vi "Main Loop.vi"(8 "error in (no error)":errorcluster, 10 "Chart Notifier":refnum<notifier>, 11 "Message Queues":T1) -> (0 "error out":errorcluster)   [LabVIEW 2018, in "Pump Module.lvlib" / "Pump Module Engine.lvlib"]
uses:
  Pump Module Engine.lvlib
  All Message Queues.ctl
  support/Message Queue/Message Cluster.ctl
  State Cluster.ctl
  State Enum.ctl
  Pump Module Settings Cluster.ctl
  Measure Instrument/PID 2 Output Enum.ctl
  Ismatec ISM 831C/Controls/Ismatech ISM831C Settings Cluster.ctl
  Ismatec 78001/Ismatec 4083.ctl
  Masterflex 7550-30/Controls/Settings Cluster.ctl
  VICI M50 Party Mode/Settings Cluster.ctl
  Tacmina QI/Tacmina QI DAQ Setting.ctl
  KNF Pump/Settings Cluster plus SIMDOS.ctl
  ASIA Pump/Pump Settings.ctl
  FLOM Pump/Settings Cluster.ctl
  SSI PR Class/SSI PR or LD Settings Cluster.ctl
  Masterflex 75211/Masterflex 75211 DAQ Setting.ctl
  Pump Module Display.ctl
  <vilib>/Platform/TimedLoop/XDataNode/timing_clust.ctl
  <vilib>/Platform/TimedLoop/XDataNode/nitl_modes.ctl
  <vilib>/Platform/TimedLoop/XDataNode/wakeup.ctl
  Tag VIs/Tag FGV Operation Enum.ctl
  support/Message Queue/Enqueue Message (Single).vi
  <vilib>/Platform/TimedLoop/XDataNode/XDataNode.xnode
  support/Message Queue/Message Queue.lvlib
  <vilib>/Platform/TimedLoop/XDataNode/XDNodeRunTimeDep.lvlib
  Pump Module.lvlib
  Ismatec ISM 831C/Ismatec ISM 831C.lvlib
  Masterflex 7550-30/Masterflex 7550-30.lvlib
  Shared Variables/Dynamic Shared Variables.lvlib
  Tacmina QI/Tacmina QI.lvlib
  KNF Pump/KNF SIMDOS.lvlib
  ASIA Pump.lvlib
  VICI M50 Party Mode/VICI M6 M50 Party Mode.lvlib
  FLOM Pump/FLOM Pump.lvlib
  SSI PR Class/SSI PR or LD Pump.lvlib
  support/Support Library.lvlib
  Masterflex 75211/Masterflex 75211.lvlib
  Ismatec 78001/Ismatec 4308.lvlib
  Program Files (x86)/Pfizer/FAST/data/AsiaPumpInterface.dll
panel:
  out "error out 2":errorcluster
  out "Period (s)":dbl format="%_4g"
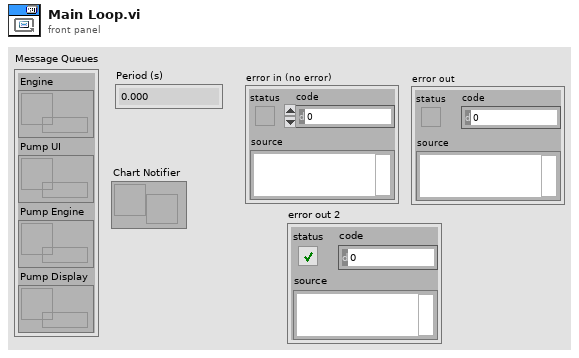
[diagram p1: front panel]
types:
  T1 = typedef "Pump Module.lvlib/All Message Queues.ctl" = cluster{"Engine":refnum<queue>, "Pump UI":refnum<queue>, "Pump Engine":refnum<queue>, "Pump Display":refnum<queue>}
  T2 = typedef "Pump Module.lvlib/Pump Module Display.ctl" = cluster{"Pump On?":enum16{"Off", "On", "Not Initialized"}, "Cycle Period":dbl, "Current Pump Speed":dbl, "Current Pump Pressure":dbl, "Current Pump Flow":dbl, "Totalized":dbl, "Output":T3}
  T3 = typedef "PID 2 Output Enum.ctl" = enum16{"Default", "Ismatec ISM 4308", "Ismatec ISM 831C", "Masterflex 7550-30", "VICI M6", "VICI M50", "Tacmina QI", "KNF SIMDOS", "ASIA Type C", "FLOM UI-22-11", "SSI PR/LD", "SSI P40", "Masterflex 75211-70"}
  T4 = typedef "XDNodeRunTimeDep.lvlib/timing_clust.ctl" = cluster{"Expected End [f-1]":u64, "Actual End [f-1]":u64, "Finished Late? [f-1]":bool, "Expected End [i-1]":u64, "Actual End [i-1]":u64, "Finished Late? [i-1]":bool, "Expected Start [i]":u64, "Actual Start [i]":u64, "Expected Start [f]":u64, "Actual Start [f]":u64, "Source Name":string, "Structure Name":string, "Period":i64, "Deadline":i64, "Offset":i64, "Start":i64, "Priority":i32, "Timeout":i32, "Mode":T5, "Wakeup Reason":T6, "Error":errorcluster, "Source Type":string, "Secondary Source Type":string, "Global End Time":u64, "Global Start Time":u64, "Frame Duration":u64, "Iteration Duration":u64, "Assigned CPU":i32, "I/O Scan Engine Mode":u32}
  T5 = typedef "XDNodeRunTimeDep.lvlib/nitl_modes.ctl" = enum32{"No Change", "Process missed periods, maintain original phase", "Discard missed periods, maintain original phase", "Process missed periods, ignore original phase", "Discard missed periods, ignore original phase"}
  T6 = typedef "XDNodeRunTimeDep.lvlib/wakeup.ctl" = enum32{"Normal", "Aborted", "Asynchronous wakeup", "Timing source error", "Timed loop error", "Timeout"}
  T7 = cluster{"enable? (F)":bool, "name":string, "alarm on":bool, "priority":u32, "ack type":enum16{"Auto", "User", "None", "Each Occurrence"}, "area":string, "description":string, "log? (T)":bool}
  T8 = typedef "Tag FGV Operation Enum.ctl" = enum16{"Init", "Set Notification Queue", "Create Tag", "Commit", "Write Tag (Numeric)", "Write Tag (Boolean)", "Read All Tags", "Read One Tag", "Delete Tag Category", "Set Alarm Parameters (Numeric)", "Set Alarm Parameters (Boolean)", "Enable All Alarms", "Disable All Alarms", "Delete All Tags", "Read Alarms", "Ack Alarm", "Read Alarm Parameters (Numeric)", "Read Alarm Parameters (Boolean)"}
  T9 = enum32{"u32BitField", "bool", "double", "string", "int8", "uint8", "int16", "uint16", "int32", "uint32", "int64", "uint64", "single", "double waveform", "int16 waveform", "array of boolean", "array of int8", "array of uint8", "array of int16", "array of uint16", "array of int32", "array of uint32", "array of int64", "array of uint64", "array of single", "array of double", "array of double waveform", "array of int16 waveform", "array of string", "variant", "timestamp", "fixed point", "custom"}
  T10 = typedef "Pump Module.lvlib/Pump Module Engine.lvlib/State Enum.ctl" = enum16{"Measuring", "Idle", "Paused"}
  T11 = typedef "Pump Module.lvlib/Pump Module Engine.lvlib/State Cluster.ctl" = cluster{"State":T10, "Start Time":timestamp, "Configuration":T12, "Current Time":timestamp, "First Iteration":bool, "Data":cluster{"Pump Speed":dbl, "Pump Pressure":dbl, "Pump Flow":dbl, "Totalized":dbl}, "Process Name":string, "Pump On?":enum16{"Off", "On", "Not Initialized"}, "Output Error":bool, "Log Started":bool, "Overpressure Alarming":bool}
  T12 = typedef "Pump Module.lvlib/Pump Module Settings Cluster.ctl" = cluster{"Cycle Period":dbl, "Manual Entry":dbl, "Output Device":T3, "Ismatech":T13, "Ismatech 3 Channel Settings":T14, "Masterflex":T15, "VICI Settings":T16, "Tacmina Settings":T17, "KNF SIMDOS Settings":T18, "ASIA Pump C":T19, "FLOM Settings":T20, "SSI PR/LD Settings":T21, "SSI P40 Settings":T21, "Masterflex 75211 Settings":T22, "Pump Calibration File":path, "Calibration Slope":dbl, "Calibration Y Intercept":dbl, "Pump Cal Enum":u16, "Reset Totalizer":bool}
  T13 = typedef "Ismatec ISM 831C.lvlib/Ismatech ISM831C Settings Cluster.ctl" = cluster{"VISA resource name":refnum<visa-resource-name>, "Simulated?":bool, "Pump Number":dbl, "Reverse?":bool}
  T14 = typedef "Ismatec 4308.lvlib/Ismatec 4083.ctl" = cluster{"VISA resource name":refnum<visa-resource-name>, "Pump Number":i16, "Channel Number":i16, "Simulated?":bool, "Reverse?":bool}
  T15 = typedef "Masterflex 7550-30.lvlib/Settings Cluster.ctl" = cluster{"VISA resource name":refnum<visa-resource-name>, "Simulated?":bool, "Pump Number":dbl, "Reverse?":bool}
  T16 = typedef "VICI M6 M50 Party Mode.lvlib/Settings Cluster.ctl" = cluster{"VISA resource name":refnum<visa-resource-name>, "Pump ID":string, "Pump Head Vol":dbl, "Reverse?":bool, "Simulated?":bool}
  T17 = typedef "Tacmina QI.lvlib/Tacmina QI DAQ Setting.ctl" = cluster{"Analog DAQ Task":refnum<k21>, "Digital DAQ Task":refnum<k21>}
  T18 = typedef "KNF SIMDOS.lvlib/Settings Cluster plus SIMDOS.ctl" = cluster{"VISA resource name":refnum<visa-resource-name>, "Simulated?":bool}
  T19 = typedef "ASIA Pump.lvlib/Pump Settings.ctl" = cluster{"ASIA Pump #":i32, "channel":i32, "Simulated":bool}
  T20 = typedef "FLOM Pump.lvlib/Settings Cluster.ctl" = cluster{"VISA resource name":refnum<visa-resource-name>, "Simulated?":bool, "Pump Number":dbl}
  T21 = typedef "SSI PR or LD Pump.lvlib/SSI PR or LD Settings Cluster.ctl" = cluster{"VISA resource name":refnum<visa-resource-name>, "Simulated?":bool}
  T22 = typedef "Masterflex 75211.lvlib/Masterflex 75211 DAQ Setting.ctl" = cluster{"Analog DAQ Task":refnum<k21>, "Digital DAQ Task":refnum<k21>}
  T23 = enum16{"Error", "Uninitialised", "Initialising", "Idle", "Filling", "Full", "Emptying", "Empty", "Pumping", "Default"}
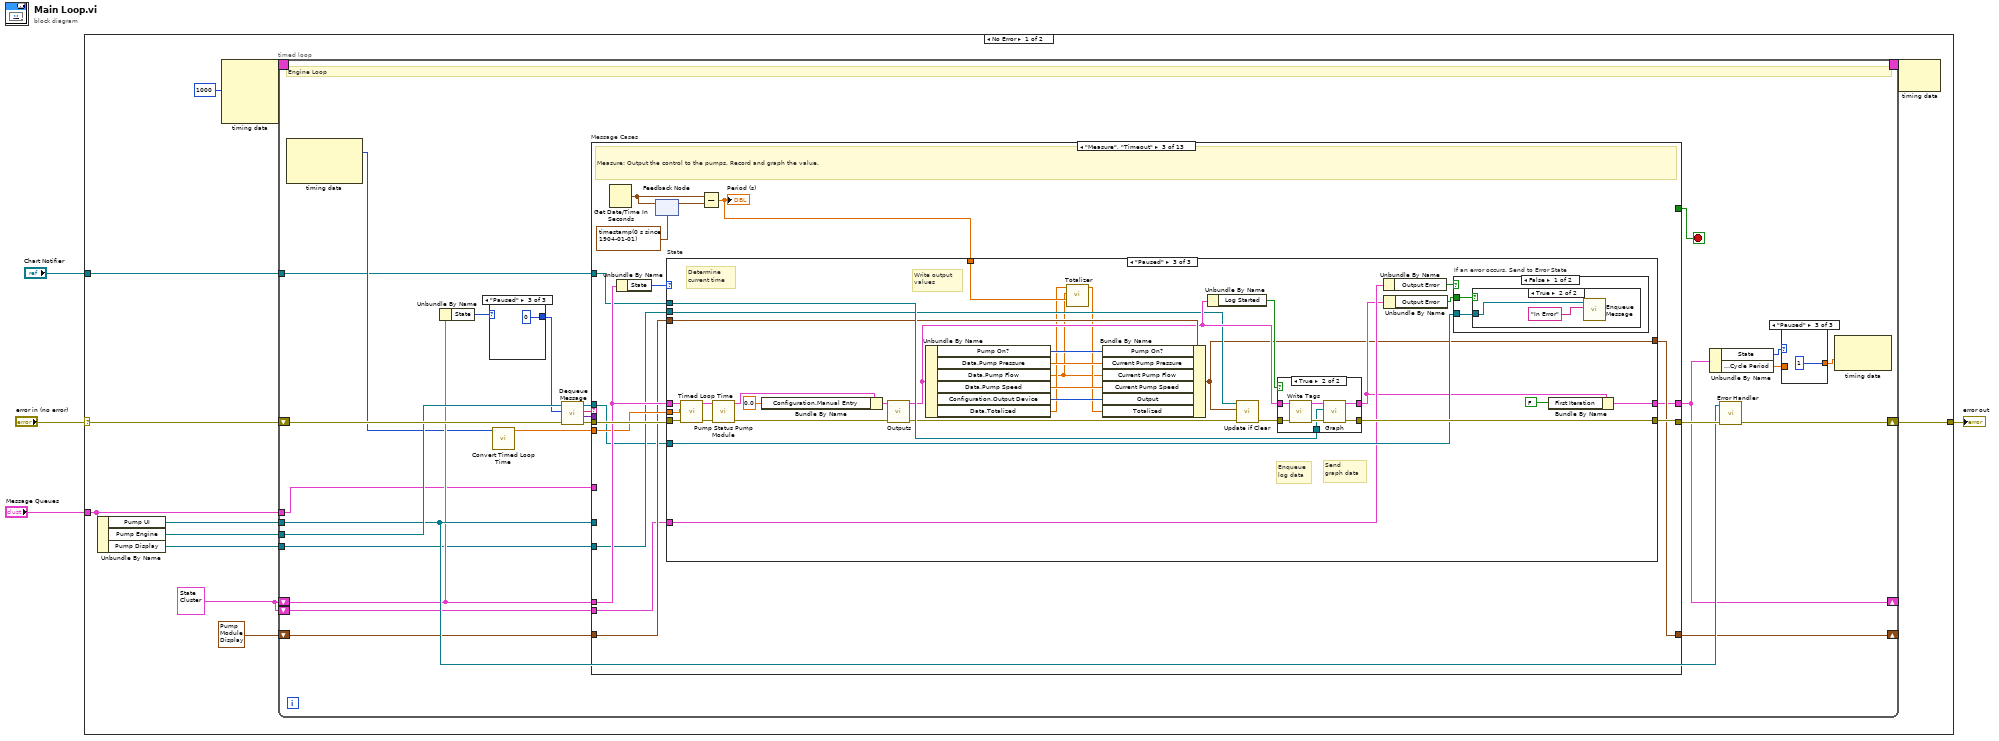
[diagram p0: block diagram]
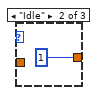
[diagram p3: hidden frame]
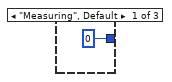
[diagram p4: hidden frame]
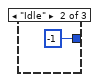
[diagram p5: hidden frame]
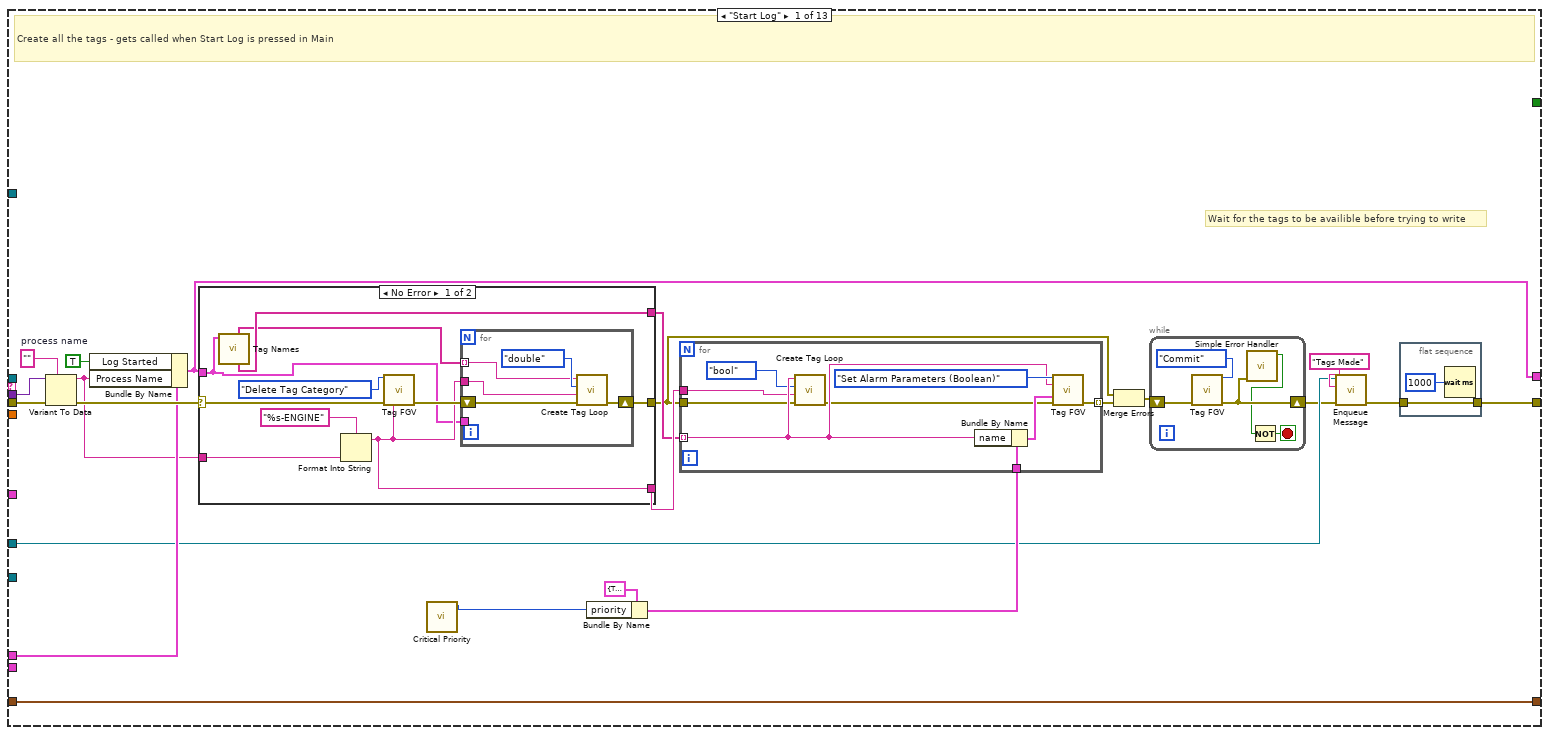
[diagram p6: hidden frame]
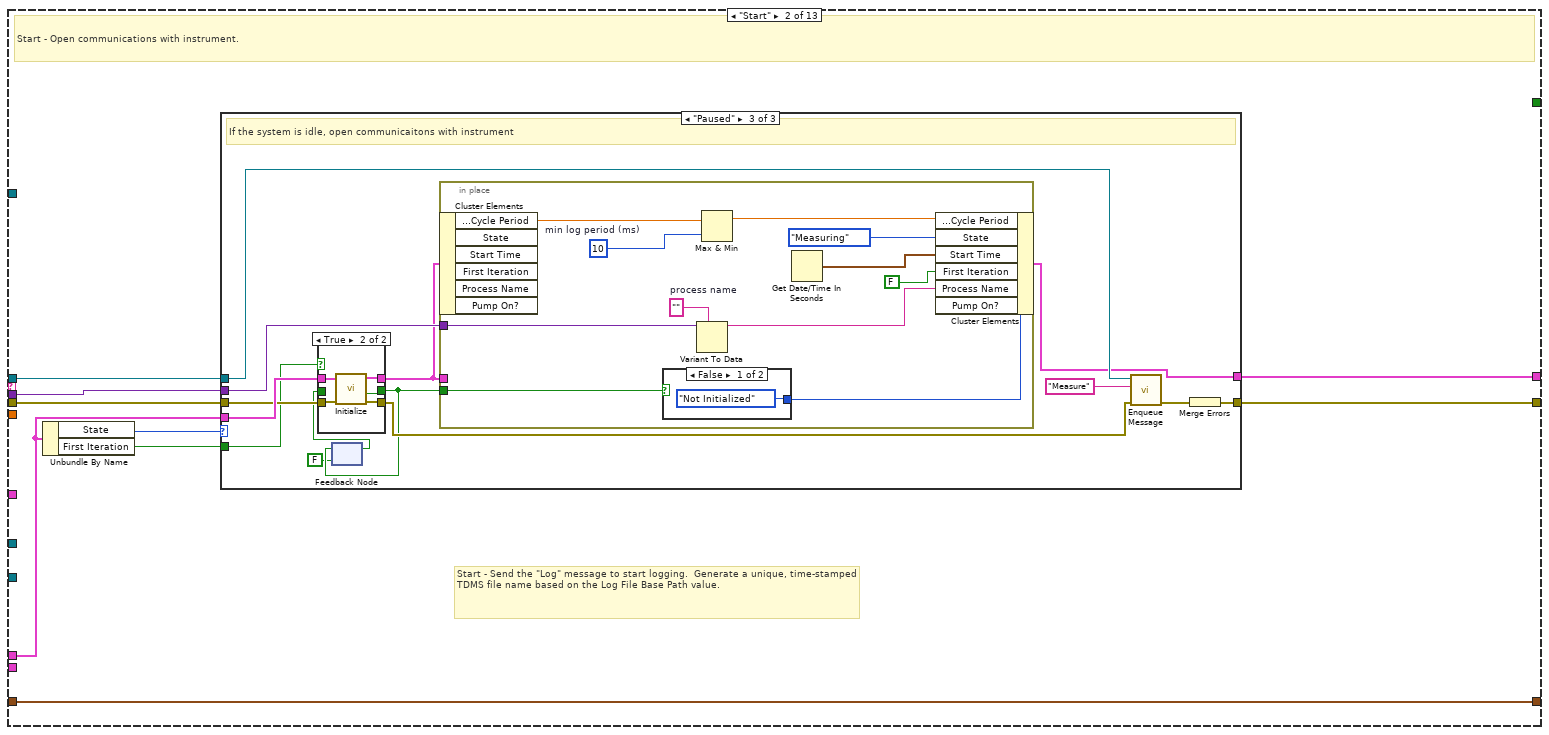
[diagram p8: hidden frame]
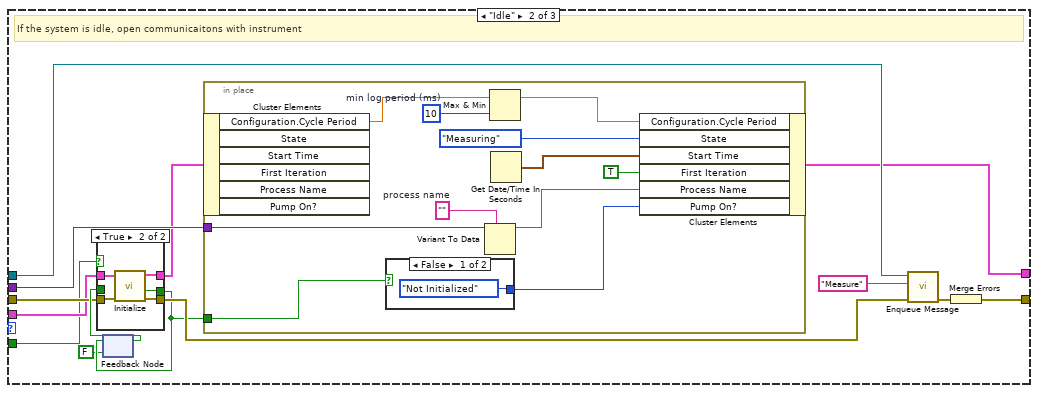
[diagram p10: hidden frame]
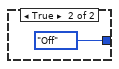
[diagram p11: hidden frame]
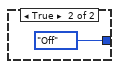
[diagram p13: hidden frame]
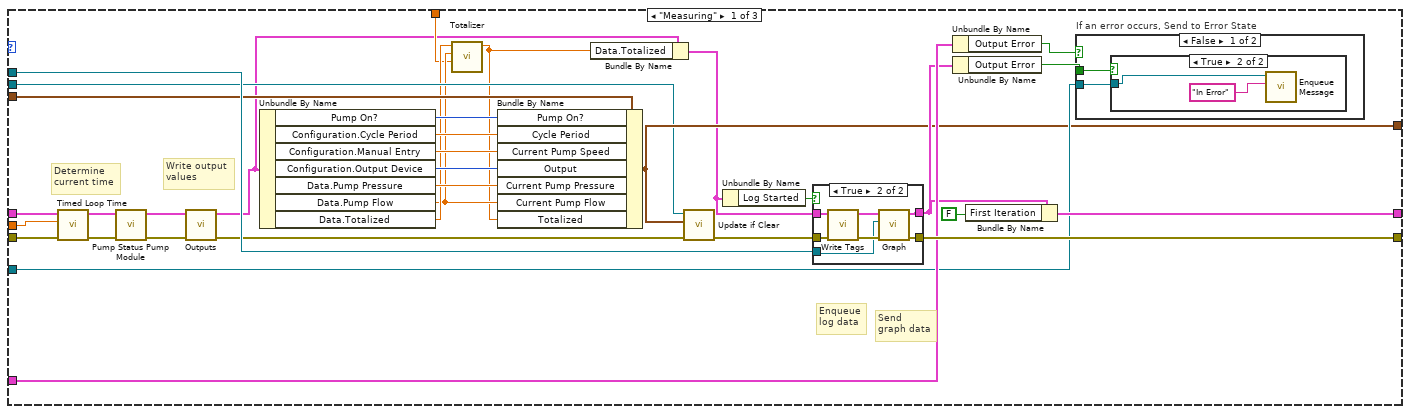
[diagram p15: hidden frame]
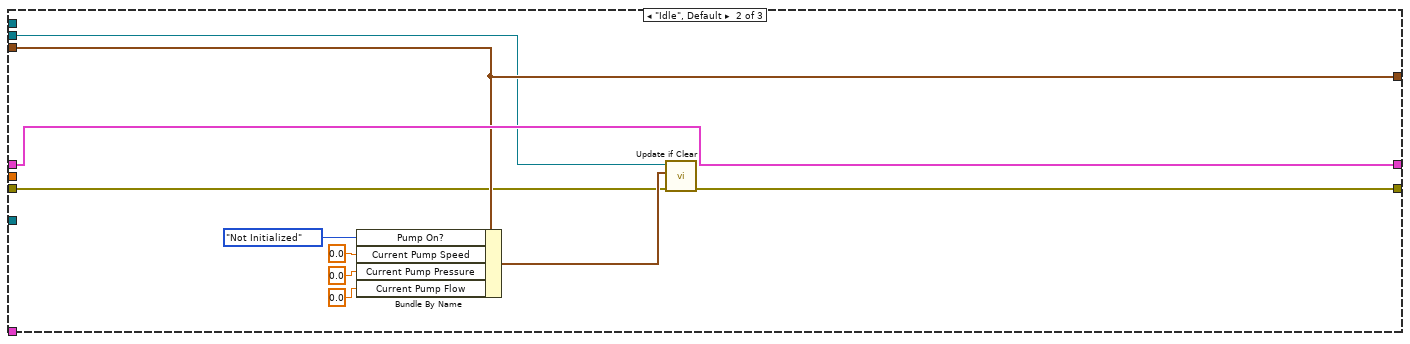
[diagram p19: hidden frame]
diagram:
  n1 = case shown="No Error" "error in (no error)" {
    selector: "error in (no error)" -> [w15 w512]
    tunnel: "Message Queues" -> [w11 _]
    tunnel: [w16 w512] -> w3
    tunnel: "Chart Notifier" -> [w9 _]
    frame No Error {
      w6 = T11 {"State"=enum."Idle", "Start Time"=timestamp(0 s since 1904-01-01), "Configuration"={"Cycle Period"=0.0, "Manual Entry"=0.0, "Output Device"=enum."VICI M6", "Ismatech"={"VISA resource name"="", "Simulated?"=FALSE, "Pump Number"=1.0, "Reverse?"=FALSE}, "Ismatech 3 Channel Settings"={"VISA resource name"="", "Pump Number"=1, "Channel Number"=0, "Simulated?"=TRUE, "Reverse?"=FALSE}, "Masterflex"={"VISA resource name"="", "Simulated?"=FALSE, "Pump Number"=1.0, "Reverse?"=FALSE}, "VICI Settings"={"VISA resource name"="", "Pump ID"="", "Pump Head Vol"=0.0, "Reverse?"=FALSE, "Simulated?"=FALSE}, "Tacmina Settings"={"Analog DAQ Task"="", "Digital DAQ Task"=""}, "KNF SIMDOS Settings"={"VISA resource name"="", "Simulated?"=TRUE}, "ASIA Pump C"={"ASIA Pump #"=0, "channel"=0, "Simulated"=FALSE}, "FLOM Settings"={"VISA resource name"="", "Simulated?"=TRUE, "Pump Number"=0.0}, "SSI PR/LD Settings"={"VISA resource name"="", "Simulated?"=FALSE}, "SSI P40 Settings"={"VISA resource name"="", "Simulated?"=FALSE}, "Masterflex 75211 Settings"={"Analog DAQ Task"="", "Digital DAQ Task"=""}, "Pump Calibration File"=path "", "Calibration Slope"=0.0, "Calibration Y Intercept"=0.0, "Pump Cal Enum"=0, "Reset Totalizer"=FALSE}, "Current Time"=timestamp(0 s since 1904-01-01), "First Iteration"=FALSE, "Data"={"Pump Speed"=0.0, "Pump Pressure"=0.0, "Pump Flow"=0.0, "Totalized"=0.0}, "Process Name"="", "Pump On?"=enum."Off", "Output Error"=FALSE, "Log Started"=FALSE, "Overpressure Alarming"=FALSE}
      n2 = Unbundle By Name(w11) -> ("Pump UI"=w14:refnum<queue>, "Pump Engine"=w10:refnum<queue>, "Pump Display"=w8:refnum<queue>)
      n3 = node-c288(i64 1000 ("Period")) -> (w13:T4)  [unwired: 3 in]
      n4 = timed-loop {
        tunnel: w10 -> [w35]
        shift-right: [w17] -> _
        shift-left: w6 -> [w31]
        shift-right: [w33] -> w16
        shift-left: w15 -> [w40]
        tunnel: w14 -> [w32]
        timing: w13 -> [_]
        timing-out: [_] -> w12
        tunnel: w11 -> [w23]
        tunnel: w9 -> [w22]
        tunnel: w8 -> [w21]
        shift-right: [w20] -> _
        shift-left: T2 {"Pump On?"=enum."Off", "Cycle Period"=500.0, "Current Pump Speed"=0.0, "Current Pump Pressure"=0.0, "Current Pump Flow"=0.0, "Totalized"=0.0, "Output"=enum."Default"} ("PM Display") -> [w19]
        shift-left: w6 -> [w18]
        stop <- w41 stop-if-true
        # "Engine Loop"
        n5 = node-c288() -> (w25:i64)  [unwired: 1 in, 2 out]
        n6 = Unbundle By Name(w31) -> ("State"=w30:T10)
        n7 = case shown="\"Paused\"" w30 {
          tunnel: [0 ("timeout in ms (-1)") -1 ("timeout in ms (-1)") 0 ("timeout in ms (-1)")] -> w29
          frame "Measuring", Default {
          }
          frame "Idle" {
          }
          frame "Paused" {
          }
        }
        n8 = call "Convert Timed Loop Time.vi"("Actual Start [i]"=w25) -> ("ET since start (s)"=w24:dbl)  [unwired: 10 in]
        n9 = call "Dequeue Message.vi"("error in (no error)"=w40, "timeout in ms (-1)"=w29, "Message Queue"=w35) -> ("error out"=w39:errorcluster, "Message Data"=w37:variant, "Message"=w38:string, "dup Message Queue"=w36:refnum<queue>)  [unwired: 5 in]
        n10 = case "Message Cases" shown="\"Measure\", \"Timeout\"" w38 {
          selector: w38 -> [_ _ _ _ _ _ _ _ _ _ _ _ w501]
          tunnel: w36 -> [_ w114 w192 _ _ _ w372 _ w387 _ _ _ _]
          tunnel: w39 -> [w58 w113 w201 w311 w337 w362 w375 w382 w401 w419 w423 w472 _]
          tunnel: [w54 w115 w202 w306 w333 w358 w377 w381 w396 w418 w429 w465 w500] -> w34
          tunnel: w31 -> [w64 w110 w200 w313 w338 w359 w368 w379 w400 w416 w425 w466 w506]
          tunnel: [w60 w107 w190 w312 w340 w354 w368 w379 w397 w414 w425 w466 w506] -> w17
          tunnel: [_ _ _ _ _ _ TRUE _ _ _ _ _ _] -> w41
          tunnel: w37 -> [w73 w111 _ _ _ w363 _ _ _ _ _ _ _]
          tunnel: w32 -> [w61 _ _ w315 _ _ w376 _ _ _ _ _ _]
          tunnel: w24 -> [_ _ w199 _ _ _ _ _ _ _ _ _ _]
          tunnel: w23 -> [_ _ _ _ _ _ _ _ _ _ _ _ _]
          tunnel: w22 -> [_ _ w196 _ _ _ _ _ _ _ _ _ _]
          tunnel: w21 -> [_ _ w195 w309 w335 _ _ _ w386 _ _ _ _]
          tunnel: w19 -> [w74 w109 w194 w308 w334 w360 w369 w380 w394 w417 w431 w475 w507]
          tunnel: [w74 w109 w193 w308 w334 w360 w369 w380 w385 w417 w431 w475 w507] -> w20
          tunnel: w18 -> [_ _ w191 _ _ _ _ _ _ _ _ _ _]
          frame "Start Log" {
            w72 = ""  # process name
            # "Wait for the tags to be availible before trying to write"
            # "Create all the tags - gets called when Start Log is pressed in Main"
            n11 = Variant To Data(error in=w58, type=w72, Variant=w73) -> (data=w59:string, error out=w71:errorcluster)
            n12 = Bundle By Name(cluster=w64, "Log Started"=TRUE, "Process Name"=w59) -> (w60:T11)
            n13 = case shown="No Error" w71 {
              selector: w71 -> [w97 w106]
              tunnel: [w100 w106] -> w53
              tunnel: [w95 _] -> w67
              tunnel: [w94 _] -> w66
              tunnel: w60 -> [w91 _]
              tunnel: w59 -> [w93 _]
              frame No Error {
                n14 = call "Tag Names.vi"("State In"=w91) -> ("All Boolean Tags"=w94:string[], "All  Numeric Tags"=w92:string[])  [unwired: 8 in, 1 out]
                n15 = Format Into String(format string="%s-ENGINE", w93) -> (resulting string=w95:string)  [unwired: 2 in, 1 out]
                n16 = call "Tag FGV.vi"("Operation"=Tag_FGV_Operation_Enum."Delete Tag Category", "error in (no error)"=w97, "Tag Category"=w95) -> ("error out"=w96:errorcluster)  [unwired: 5 in, 7 out]
                n17 = for {
                  shift-right: [w101] -> w100
                  shift-left: w96 -> [w102]
                  tunnel: w95 -> [w103]
                  tunnel: w92 -> [w104] mode=indexing
                  tunnel: w91 -> [_]
                  n18 = call "Create Tag Loop.vi"("error in (no error)"=w102, "Tag Category"=w103, "data type"=T9."double", "Tag Name"=w104) -> ("error out"=w101:errorcluster)  [unwired: 7 in]
                }
              }
              frame Error {
              }
            }
            n19 = call "Critical Priority.vi"() -> ("critical priority"=w70:i32)  [unwired: 11 in]
            n20 = Bundle By Name(cluster=T7 {"enable? (F)"=TRUE, "name"="Boolean", "alarm on"=TRUE, "priority"=1, "ack type"=enum."Each Occurrence", "area"="a", "description"="", "log? (T)"=TRUE} ("Boolean alarm settings"), "priority"=w70) -> (w68:T7)
            n21 = for {
              tunnel: w68 -> [w90]
              tunnel: [w89] -> w65 mode=indexing
              tunnel: w66 -> [w86] mode=indexing
              tunnel: w53 -> [w83]
              tunnel: w67 -> [w84]
              n22 = call "Create Tag Loop.vi"("error in (no error)"=w83, "Tag Category"=w84, "data type"=T9."bool", "Tag Name"=w86) -> ("error out"=w82:errorcluster)  [unwired: 7 in]
              n23 = Bundle By Name(cluster=w90, "name"=w86) -> (w88:T7)
              n24 = call "Tag FGV.vi"("Operation"=Tag_FGV_Operation_Enum."Set Alarm Parameters (Boolean)", "Tag Name"=w86, "Data"=w88, "error in (no error)"=w82) -> ("error out"=w89:errorcluster)  [unwired: 4 in, 7 out]
            }
            n25 = Merge Errors(w53, w65) -> (w57:errorcluster)
            n26 = while {
              shift-right: [w79] -> w56
              shift-left: w57 -> [w80]
              stop <- w77 stop-if-true
              n27 = call "Tag FGV.vi"("Operation"=Tag_FGV_Operation_Enum."Commit", "error in (no error)"=w80) -> ("error out"=w79:errorcluster)  [unwired: 6 in, 7 out]
              n28 = call <vilib>:"Simple Error Handler.vi"("error in (no error)"=w79) -> ("error?"=w78:bool)  [unwired: 4 in, 4 out]
              n29 = Not(x=w78) -> (.not. x?=w77:bool)
            }
            n30 = call-poly "Enqueue Message.vi"("error in (no error)"=w56, "Message"="Tags Made", "Message Queue"=w61) -> ("error out"=w55:errorcluster)  [unwired: 7 in, 1 out]
            n31 = flat-sequence {
              tunnel: [w75] -> w54
              tunnel: w55 -> [w75]
              frame #0 {
                n32 = Wait (ms)(milliseconds to wait=u32 1000) -> ()  [unwired: 1 out]
              }
            }
          }
          frame "Start" {
            # "Start - Send the \"Log\" message to start logging.  Generate a unique, time-stamped TDMS file name based on the Log File Base Path value."
            # "Start - Open communications with instrument."
            n33 = Unbundle By Name(w110) -> ("State"=w112:T10, "First Iteration"=w108:bool)
            n34 = case shown="\"Paused\"" w112 {
              tunnel: [w116 w131 w166] -> w115
              tunnel: w114 -> [_ w128 w163]
              tunnel: w113 -> [w116 w125 w160]
              tunnel: w110 -> [w117 w124 w161]
              tunnel: [w117 w119 w154] -> w107
              tunnel: w111 -> [_ w127 w162]
              tunnel: w108 -> [_ w121 w156]
              frame "Measuring", Default {
                # "The system is already running. Ignore the \"Start\" message."
              }
              frame "Idle" {
                # "If the system is idle, open communicaitons with instrument"
                n35 = feedback #1(FALSE ("Initialized")) -> (w126:bool)
                n36 = case shown="True" w121 {
                  tunnel: w125 -> [w146 w151]
                  tunnel: w124 -> [w147 w152]
                  tunnel: [w147 w150] -> w120
                  tunnel: [w146 w148] -> w123
                  tunnel: [w145 w149] -> w122
                  tunnel: w126 -> [w145 _]
                  frame False {
                  }
                  frame True {
                    n37 = call "Initialize.vi"("error in (no error)"=w151, "State in"=w152) -> ("error out"=w148:errorcluster, "Initialized"=w149:bool, "State out"=w150:T11)  [unwired: 7 in]
                  }
                }
                n38 = feedback-in #1(w122) -> ()
                n39 = in-place {
                  in-place-border: w127 -> [w140]
                  in-place-border: w122 -> [w139]
                  w141 = ""  # process name
                  w142 = 10  # min log period (ms)
                  n40 = in-place-cluster #2(w120) -> ("Configuration.Cycle Period"=w138:dbl)  [unwired: 5 out]
                  n41 = case shown="False" w139 {
                    tunnel: [enum16{"Off", "On", "Not Initialized"}."Not Initialized" ("Pump On?") enum16{"Off", "On", "Not Initialized"}."Off" ("Pump On?")] -> w132
                    frame False {
                    }
                    frame True {
                    }
                  }
                  n42 = Variant To Data(type=w141, Variant=w140) -> (data=w133:string)  [unwired: 1 in, 1 out]
                  n43 = Max & Min(x=w138, y=w142) -> (max(x,y)=w137:dbl)  [unwired: 1 out]
                  n44 = Get Date/Time In Seconds() -> (seconds since 1Jan1904=w135:timestamp)
                  n45 = in-place-cluster #2("Configuration.Cycle Period"=w137, "State"=State_Enum."Measuring", "Start Time"=w135, "First Iteration"=TRUE, "Process Name"=w133, "Pump On?"=w132) -> (w119:T11)
                }
                n46 = call-poly "Enqueue Message.vi"("error in (no error)"=w123, "Message"="Measure", "Message Queue"=w128) -> ("error out"=w129:errorcluster)  [unwired: 7 in, 1 out]
                n47 = Merge Errors(w129) -> (w131:errorcluster)
              }
              frame "Paused" {
                # "If the system is idle, open communicaitons with instrument"
                n48 = feedback #3(FALSE ("Initialized")) -> (w157:bool)
                n49 = case shown="True" w156 {
                  tunnel: w160 -> [w181 w186]
                  tunnel: w161 -> [w182 w187]
                  tunnel: [w182 w185] -> w155
                  tunnel: [w181 w183] -> w159
                  tunnel: [w180 w184] -> w158
                  tunnel: w157 -> [w180 _]
                  frame False {
                  }
                  frame True {
                    n50 = call "Initialize.vi"("error in (no error)"=w186, "State in"=w187) -> ("error out"=w183:errorcluster, "Initialized"=w184:bool, "State out"=w185:T11)  [unwired: 7 in]
                  }
                }
                n51 = feedback-in #3(w158) -> ()
                n52 = in-place {
                  in-place-border: w162 -> [w175]
                  in-place-border: w155 -> [_]
                  in-place-border: w158 -> [w174]
                  w176 = ""  # process name
                  w177 = 10  # min log period (ms)
                  n53 = in-place-cluster #4(w155) -> ("Configuration.Cycle Period"=w173:dbl)  [unwired: 5 out]
                  n54 = case shown="False" w174 {
                    tunnel: [enum16{"Off", "On", "Not Initialized"}."Not Initialized" ("Pump On?") enum16{"Off", "On", "Not Initialized"}."Off" ("Pump On?")] -> w167
                    frame False {
                    }
                    frame True {
                    }
                  }
                  n55 = Variant To Data(type=w176, Variant=w175) -> (data=w168:string)  [unwired: 1 in, 1 out]
                  n56 = Max & Min(x=w173, y=w177) -> (max(x,y)=w172:dbl)  [unwired: 1 out]
                  n57 = Get Date/Time In Seconds() -> (seconds since 1Jan1904=w170:timestamp)
                  n58 = in-place-cluster #4("Configuration.Cycle Period"=w172, "State"=State_Enum."Measuring", "Start Time"=w170, "First Iteration"=FALSE, "Process Name"=w168, "Pump On?"=w167) -> (w154:T11)
                }
                n59 = call-poly "Enqueue Message.vi"("error in (no error)"=w159, "Message"="Measure", "Message Queue"=w163) -> ("error out"=w164:errorcluster)  [unwired: 7 in, 1 out]
                n60 = Merge Errors(w164) -> (w166:errorcluster)
              }
            }
          }
          frame "Measure", "Timeout" {
            # "Measure: Output the control to the pumps. Record and graph the value."
            n61 = Get Date/Time In Seconds() -> (seconds since 1Jan1904=w197:timestamp)
            n62 = Unbundle By Name(w200) -> ("State"=w203:T10)
            n63 = feedback-in #5(w197) -> ()
            n64 = feedback #5(timestamp(0 s since 1904-01-01) ("seconds since 1Jan1904")) -> (w198:timestamp)
            n65 = Subtract(x=w197, y=w198) -> (x-y=w188:dbl)
            "Period (s)" <- w188
            n66 = case "State" shown="\"Paused\"" w203 {
              tunnel: w201 -> [w235 w251 w286]
              tunnel: w200 -> [w234 w259 w287]
              tunnel: [w236 w250 w281] -> w202
              tunnel: [w232 w259 w272] -> w190
              tunnel: w199 -> [w233 _ w291]
              tunnel: w196 -> [w230 _ w292]
              tunnel: w195 -> [w210 w253 w267]
              tunnel: w194 -> [w227 w258 w290]
              tunnel: [w213 w258 w266] -> w193
              tunnel: w192 -> [w216 _ w278]
              tunnel: w191 -> [w218 _ w276]
              tunnel: w188 -> [w207 _ w263]
              frame "Measuring" {
                # "Determine\ncurrent time"
                # "Send\ngraph data"
                # "Enqueue\nlog data"
                # "Write output\nvalues"
                n67 = call "Timed Loop Time.vi"("error in (no error)"=w235, "ET since start (s)"=w233, "State in"=w234) -> ("error out"=w225:errorcluster, "State out"=w224:T11)  [unwired: 7 in]
                n68 = call "Pump Status Pump Module.vi"("error in (no error)"=w225, 11:w224) -> ("error out"=w228:errorcluster, "State out"=w229:T11)  [unwired: 8 in]
                n69 = call "Outputs.vi"("error in (no error)"=w228, "State in"=w229) -> ("error out"=w212:errorcluster, "State out"=w206:T11)  [unwired: 8 in]
                n70 = Unbundle By Name(w206) -> ("Pump On?"=w226:enum16{"Off", "On", "Not Initialized"}, "Configuration.Cycle Period"=w223:dbl, "Configuration.Manual Entry"=w222:dbl, "Configuration.Output Device"=w215:T3, "Data.Pump Pressure"=w214:dbl, "Data.Pump Flow"=w208:dbl, "Data.Totalized"=w209:dbl)
                n71 = call "Totalizer.vi"("Period"=w207, "Flow Rate"=w208, "Current Total"=w209) -> ("New Total"=w204:dbl)  [unwired: 8 in]
                n72 = Bundle By Name(cluster=w227, "Pump On?"=w226, "Cycle Period"=w223, "Current Pump Speed"=w222, "Output"=w215, "Current Pump Pressure"=w214, "Current Pump Flow"=w208, "Totalized"=w204) -> (w213:T2)
                n73 = Bundle By Name(cluster=w206, "Data.Totalized"=w204) -> (w205:T11)
                n74 = call "Update if Clear.vi"("error in (no error)"=w212, "Message Data"=w213, "Queue in"=w210) -> ("error out"=w211:errorcluster)  [unwired: 8 in]
                n75 = Unbundle By Name(w205) -> ("Log Started"=w221:bool)
                n76 = case shown="True" w221 {
                  tunnel: [w241 w247] -> w236
                  tunnel: [w242 w246] -> w217
                  tunnel: w230 -> [_ w245]
                  tunnel: w205 -> [w242 w244]
                  tunnel: w211 -> [w241 w243]
                  frame False {
                  }
                  frame True {
                    n77 = call "Write Tags.vi"("error in (no error)"=w243, "State in"=w244) -> ("error out"=w248:errorcluster, "State out"=w249:T11)  [unwired: 8 in]
                    n78 = call "Graph.vi"("error in (no error)"=w248, "notifier out"=w245, "State in"=w249) -> ("error out"=w247:errorcluster, "State out"=w246:T11)  [unwired: 7 in]
                  }
                }
                n79 = Unbundle By Name(w218) -> ("Output Error"=w219:bool)
                n80 = Unbundle By Name(w217) -> ("Output Error"=w220:bool)
                n81 = Bundle By Name(cluster=w217, "First Iteration"=FALSE) -> (w232:T11)
                n82 = case "If an error occurs, Send to Error State" shown="False" w219 {
                  tunnel: w220 -> [w238 _]
                  tunnel: w216 -> [w237 _]
                  frame False {
                    n83 = case shown="True" w238 {
                      tunnel: w237 -> [_ w239]
                      frame False {
                      }
                      frame True {
                        n84 = call-poly "Enqueue Message.vi"("Message"="In Error", "Message Queue"=w239) -> ()  [unwired: 8 in, 2 out]
                      }
                    }
                  }
                  frame True {
                  }
                }
              }
              frame "Idle", Default {
                n85 = Bundle By Name(cluster=w258, "Pump On?"=enum16{"Off", "On", "Not Initialized"}."Not Initialized", "Current Pump Speed"=0.0, "Current Pump Pressure"=0.0, "Current Pump Flow"=0.0) -> (w252:T2)
                n86 = call "Update if Clear.vi"("error in (no error)"=w251, "Message Data"=w252, "Queue in"=w253) -> ("error out"=w250:errorcluster)  [unwired: 8 in]
              }
              frame "Paused" {
                # "Determine\ncurrent time"
                # "Write output\nvalues"
                # "Send\ngraph data"
                # "Enqueue\nlog data"
                n87 = call "Timed Loop Time.vi"("error in (no error)"=w286, "ET since start (s)"=w291, "State in"=w287) -> ("error out"=w283:errorcluster, "State out"=w285:T11)  [unwired: 7 in]
                n88 = call "Pump Status Pump Module.vi"("error in (no error)"=w283, 11:w285) -> ("error out"=w282:errorcluster, "State out"=w284:T11)  [unwired: 8 in]
                n89 = Bundle By Name(cluster=w284, "Configuration.Manual Entry"=0.0) -> (w288:T11)
                n90 = call "Outputs.vi"("error in (no error)"=w282, "State in"=w288) -> ("error out"=w265:errorcluster, "State out"=w271:T11)  [unwired: 8 in]
                n91 = Unbundle By Name(w271) -> ("Pump On?"=w280:enum16{"Off", "On", "Not Initialized"}, "Data.Pump Pressure"=w279:dbl, "Data.Pump Flow"=w260:dbl, "Data.Pump Speed"=w269:dbl, "Configuration.Output Device"=w268:T3, "Data.Totalized"=w262:dbl)
                n92 = call "Totalizer.vi"("Period"=w263, "Flow Rate"=w260, "Current Total"=w262) -> ("New Total"=w261:dbl)  [unwired: 8 in]
                n93 = Bundle By Name(cluster=w290, "Pump On?"=w280, "Current Pump Pressure"=w279, "Current Pump Flow"=w260, "Current Pump Speed"=w269, "Output"=w268, "Totalized"=w261) -> (w266:T2)
                n94 = Unbundle By Name(w271) -> ("Log Started"=w270:bool)
                n95 = call "Update if Clear.vi"("error in (no error)"=w265, "Message Data"=w266, "Queue in"=w267) -> ("error out"=w264:errorcluster)  [unwired: 8 in]
                n96 = case shown="True" w270 {
                  tunnel: w292 -> [_ w299]
                  tunnel: w264 -> [w293 w298]
                  tunnel: [w293 w297] -> w281
                  tunnel: w271 -> [w294 w296]
                  tunnel: [w294 w295] -> w273
                  frame False {
                  }
                  frame True {
                    n97 = call "Write Tags.vi"("error in (no error)"=w298, "State in"=w296) -> ("error out"=w301:errorcluster, "State out"=w300:T11)  [unwired: 8 in]
                    n98 = call "Graph.vi"("error in (no error)"=w301, "notifier out"=w299, "State in"=w300) -> ("error out"=w297:errorcluster, "State out"=w295:T11)  [unwired: 7 in]
                  }
                }
                n99 = Unbundle By Name(w276) -> ("Output Error"=w275:bool)
                n100 = Unbundle By Name(w273) -> ("Output Error"=w277:bool)
                n101 = case "If an error occurs, Send to Error State" shown="False" w275 {
                  tunnel: w277 -> [w303 _]
                  tunnel: w278 -> [w302 _]
                  frame False {
                    n102 = case shown="True" w303 {
                      tunnel: w302 -> [_ w305]
                      frame False {
                      }
                      frame True {
                        n103 = call-poly "Enqueue Message.vi"("Message"="In Error", "Message Queue"=w305) -> ()  [unwired: 8 in, 2 out]
                      }
                    }
                  }
                  frame True {
                  }
                }
                n104 = Bundle By Name(cluster=w273, "First Iteration"=FALSE) -> (w272:T11)
              }
            }
          }
          frame "Stop" {
            # "Stop - Flush the message queue of any pending \"Log\" messages. Call 'Flush Data to Log File.vi' so any pending data is not lost."
            n105 = call <vilib>:"Clear Errors.vi"("error in (no error)"=w311) -> ("error out"=w310:errorcluster)  [unwired: 5 in, 1 out]
            n106 = Unbundle By Name(w313) -> ("State"=w314:T10)
            n107 = case shown="\"Measuring\", Default" w314 {
              tunnel: [w320 w326] -> w307
              tunnel: w310 -> [w317 w326]
              tunnel: w315 -> [w324 _]
              tunnel: w313 -> [w318 w325]
              tunnel: [w322 w325] -> w312
              frame "Measuring", Default {
                # "If the system is logging, stop logging."
                n108 = call "Close.vi"("error in (no error)"=w317, "State in"=w318) -> ("error out"=w316:errorcluster, "State out"=w319:T11)  [unwired: 7 in, 1 out]
                n109 = Bundle By Name(cluster=w319, "State"=State_Enum."Idle") -> (w322:T11)
                n110 = call-poly "Enqueue Message.vi"("error in (no error)"=w316, "Message"="Logging Stopped", "Message Queue"=w324) -> ("error out"=w320:errorcluster)  [unwired: 7 in, 1 out]
              }
              frame "Idle" {
                # "The system is already idle. Ignore the \"Stop\" message."
              }
            }
            n111 = call "Update if Clear.vi"("error in (no error)"=w307, "Message Data"=w308, "Queue in"=w309) -> ("error out"=w306:errorcluster)  [unwired: 8 in]
          }
          frame "Pause" {
            # "Stop - Flush the message queue of any pending \"Log\" messages. Call 'Flush Data to Log File.vi' so any pending data is not lost."
            n112 = Unbundle By Name(w338) -> ("First Iteration"=w339:bool)  [unwired: 1 out]
            n113 = case shown="True" w339 {
              tunnel: w338 -> [w341 w345]
              tunnel: [w341 w349] -> w336
              tunnel: w337 -> [w342 w346]
              tunnel: [w342 w347] -> w329
              frame False {
              }
              frame True {
                # "If we start on a pause condition, initialize the pump"
                n114 = call "Initialize.vi"("error in (no error)"=w346, "State in"=w345) -> ("error out"=w347:errorcluster, "Initialized"=w348:bool, "State out"=w344:T11)  [unwired: 7 in]
                n115 = case shown="True" w348 {
                  tunnel: [enum16{"Off", "On", "Not Initialized"}."Not Initialized" ("Pump On?") enum16{"Off", "On", "Not Initialized"}."Off" ("Pump On?")] -> w350
                  tunnel: [_ FALSE] -> w343
                  frame False {
                  }
                  frame True {
                  }
                }
                n116 = Bundle By Name(cluster=w344, "Pump On?"=w350, "First Iteration"=w343) -> (w349:T11)
              }
            }
            n117 = call <vilib>:"Clear Errors.vi"("error in (no error)"=w329) -> ("error out"=w330:errorcluster)  [unwired: 5 in, 1 out]
            n118 = call "Pause.vi"("error in (no error)"=w330, "State in"=w336) -> ("error out"=w328:errorcluster, "State out"=w331:T11)  [unwired: 8 in]
            n119 = Bundle By Name(cluster=w331, "State"=State_Enum."Paused") -> (w340:T11)
            n120 = Merge Errors(w328, w329) -> (w327:errorcluster)
            n121 = call "Update if Clear.vi"("error in (no error)"=w327, "Message Data"=w334, "Queue in"=w335) -> ("error out"=w333:errorcluster)  [unwired: 8 in]
          }
          frame "Update Settings" {
            w361 = T12 {"Cycle Period"=0.0, "Manual Entry"=0.0, "Output Device"=enum."VICI M6", "Ismatech"={"VISA resource name"="", "Simulated?"=FALSE, "Pump Number"=1.0, "Reverse?"=FALSE}, "Ismatech 3 Channel Settings"={"VISA resource name"="", "Pump Number"=1, "Channel Number"=0, "Simulated?"=TRUE, "Reverse?"=FALSE}, "Masterflex"={"VISA resource name"="", "Simulated?"=FALSE, "Pump Number"=1.0, "Reverse?"=FALSE}, "VICI Settings"={"VISA resource name"="", "Pump ID"="", "Pump Head Vol"=0.0, "Reverse?"=FALSE, "Simulated?"=FALSE}, "Tacmina Settings"={"Analog DAQ Task"="", "Digital DAQ Task"=""}, "KNF SIMDOS Settings"={"VISA resource name"="", "Simulated?"=TRUE}, "ASIA Pump C"={"ASIA Pump #"=0, "channel"=0, "Simulated"=FALSE}, "FLOM Settings"={"VISA resource name"="", "Simulated?"=TRUE, "Pump Number"=0.0}, "SSI PR/LD Settings"={"VISA resource name"="", "Simulated?"=FALSE}, "SSI P40 Settings"={"VISA resource name"="", "Simulated?"=FALSE}, "Masterflex 75211 Settings"={"Analog DAQ Task"="", "Digital DAQ Task"=""}, "Pump Calibration File"=path "", "Calibration Slope"=0.0, "Calibration Y Intercept"=0.0, "Pump Cal Enum"=0, "Reset Totalizer"=FALSE}  # Configuration
            # "New settings are available, update the current ones stored in the shift register with the settings sent as part of the message"
            n122 = Variant To Data(error in=w362, type=w361, Variant=w363) -> (data=w357:T12, error out=w358:errorcluster)
            n123 = Bundle By Name(cluster=w359, "Configuration"=w357) -> (w355:T11)
            n124 = Unbundle By Name(w355) -> ("Configuration.Reset Totalizer"=w356:bool)
            n125 = case shown="True" w356 {
              tunnel: w355 -> [w364 w367]
              tunnel: [w364 w365] -> w354
              frame False {
              }
              frame True {
                n126 = Bundle By Name(cluster=w367, "Data.Totalized"=0.0) -> (w365:T11)
              }
            }
          }
          frame "Exit" {
            # "Release the Logging queue reference"
            # "Don't check the error out. The UI message queue may have already been released."
            # "Stop the VI"
            # "Exit - Send the Exit message to the UI Message Handler.  Call 'Flush Data to Log File.vi' so any pending data is not lost."
            n127 = Release Queue(queue=w372, error in (no error)=w375) -> (error out=w371:errorcluster)  [unwired: 1 in, 2 out]
            n128 = call-poly "Enqueue Message.vi"("Priority Message? (F)"=TRUE, "Message"="Exit", "Message Queue"=w376) -> ("error out"=w370:errorcluster)  [unwired: 7 in, 1 out]
            n129 = call <vilib>:"Clear Errors.vi"("error in (no error)"=w370) -> ()  [unwired: 5 in, 2 out]
            n130 = Merge Errors(w371) -> (w377:errorcluster)
          }
          frame "---Copy This Frame---" {
            # "Duplicate this frame when creating new messages.  Change this comment in the duplicated frame to describe this message."
            n131 = Merge Errors(w382) -> (w381:errorcluster)
          }
          frame "In Error" {
            # "If we have a disconnect Error we will go to this state, and attempt to reconnect and get back to the pre-error state"
            n132 = Merge Errors(w401) -> (w398:errorcluster)
            n133 = call "Initialize.vi"("error in (no error)"=w398, "State in"=w400) -> ("error out"=w384:errorcluster, "Initialized"=w399:bool, "State out"=w395:T11)  [unwired: 7 in]
            n134 = Unbundle By Name(w395) -> ("Pump On?"=w388:enum16{"Off", "On", "Not Initialized"}, "Configuration.Cycle Period"=w389:dbl, "Data.Pump Speed"=w390:dbl, "Data.Pump Pressure"=w391:dbl, "Data.Pump Flow"=w392:dbl, "Configuration.Output Device"=w393:T3)
            n135 = Bundle By Name(cluster=w394, "Pump On?"=w388, "Cycle Period"=w389, "Current Pump Speed"=w390, "Current Pump Pressure"=w391, "Current Pump Flow"=w392, "Output"=w393) -> (w385:T2)
            n136 = call "Update if Clear.vi"("error in (no error)"=w384, "Message Data"=w385, "Queue in"=w386) -> ("error out"=w383:errorcluster)  [unwired: 8 in]
            n137 = case shown="False" w399 {
              tunnel: w387 -> [w406 w410]
              tunnel: w383 -> [w405 w409]
              tunnel: [w403 w412] -> w397
              tunnel: w395 -> [w403 w412]
              tunnel: [w402 w408] -> w396
              frame False {
                n138 = Wait (ms)(milliseconds to wait=u32 5000) -> ()  [unwired: 1 out]
                n139 = call-poly "Enqueue Message.vi"("error in (no error)"=w405, "Message"="In Error", "Message Queue"=w406) -> ("error out"=w402:errorcluster)  [unwired: 7 in, 1 out]
              }
              frame True {
                n140 = call-poly "Enqueue Message.vi"("error in (no error)"=w409, "Message"="Measure", "Message Queue"=w410) -> ("error out"=w408:errorcluster)  [unwired: 7 in, 1 out]
              }
            }
            "error out 2" <- w401
          }
          frame "Initialize" {
            # "Duplicate this frame when creating new messages.  Change this comment in the duplicated frame to describe this message."
            n141 = Merge Errors(w419) -> (w418:errorcluster)
            n142 = Bundle By Name(cluster=w416, "Log Started"=FALSE, "First Iteration"=TRUE) -> (w414:T11)
          }
          frame "Fill ASIA" {
            # "Duplicate this frame when creating new messages.  Change this comment in the duplicated frame to describe this message."
            n143 = Unbundle By Name(w425) -> ("Configuration.ASIA Pump C"=w420:T19)
            n144 = Unbundle By Name(w420) -> ("ASIA Pump #"=w427:i32, "channel"=w428:i32)
            n145 = call "Pump Status.vi"("ASIA Pump C Settings in"=w420, "error in (no error)"=w423) -> ("Connection Error"=w421:bool, "syringeSize (ml)"=w424:sgl, "error out"=w422:errorcluster)  [unwired: 5 in, 6 out]
            n146 = Multiply(x=w424, y=4000.0) -> (x*y=w426:dbl)
            n147 = case shown="False" w421 {
              tunnel: [w436 w463] -> w429
              tunnel: w428 -> [w441 _]
              tunnel: w427 -> [w440 _]
              tunnel: w426 -> [w439 _]
              tunnel: w422 -> [w438 w463]
              tunnel: w420 -> [w435 _]
              frame False {
                n148 = call "ASIA Reserve Pump.vi"("error in (no error)"=w438, "ASIA Pump # In"=w440) -> ("error out"=w445:errorcluster, "ASIA Pump # Out"=w444:i32)  [unwired: 8 in]
                n149 = dll-call lib="C:/Program Files (x86)/Pfizer/FAST/data/AsiaPumpInterface.dll" fn="fill"(error in=w445, "pumpNum"=w444, "channel"=w441, "rate"=w439) -> (error out=w443:errorcluster, "pumpNum"=w442:u32)  [unwired: 5 in, 1 out]
                n150 = node-c288(i64 100 ("Period")) -> (w434:T4)  [unwired: 3 in]
                n151 = call "ASIA Release Pump.vi"("error in (no error)"=w443, "pumpNum"=w442) -> ("error out"=w437:errorcluster)  [unwired: 8 in, 1 out]
                n152 = timed-loop {
                  tunnel: w437 -> [w454]
                  tunnel: [w453] -> w436
                  tunnel: w435 -> [w452]
                  timing: w434 -> [_]
                  timing-out: [_] -> w433
                  i -> [w449]
                  stop <- w447 stop-if-true
                  n153 = node-c288() -> ()  [unwired: 1 in, 1 out]
                  n154 = call "Pump Status.vi"("ASIA Pump C Settings in"=w452, "error in (no error)"=w454) -> ("PumpStatusCode"=w451:T23, "error out"=w453:errorcluster)  [unwired: 5 in, 7 out]
                  n155 = case shown="\"Error\", Default" w451 {
                    tunnel: [FALSE TRUE] -> w448
                    frame "Error", Default {
                    }
                    frame "Full" {
                    }
                  }
                  n156 = Greater?(x=w449, y=600) -> (0:w446:bool)
                  n157 = node-c288() -> ()  [unwired: 1 in, 1 out]
                  n158 = Or(x=w448, y=w446) -> (x .or. y?=w447:bool)
                }
                n159 = node-c288(w433) -> ()  [unwired: 1 out]
              }
              frame True {
              }
            }
          }
          frame "Empty ASIA" {
            # "Duplicate this frame when creating new messages.  Change this comment in the duplicated frame to describe this message."
            n160 = Unbundle By Name(w466) -> ("Configuration.ASIA Pump C"=w464:T19)
            n161 = Unbundle By Name(w464) -> ("ASIA Pump #"=w470:i32, "channel"=w469:i32)
            n162 = call "Pump Status.vi"("ASIA Pump C Settings in"=w464, "error in (no error)"=w472) -> ("Connection Error"=w468:bool, "syringeSize (ml)"=w473:sgl, "error out"=w471:errorcluster)  [unwired: 5 in, 6 out]
            n163 = Multiply(x=w473, y=4000.0) -> (x*y=w467:dbl)
            n164 = case shown="False" w468 {
              tunnel: [w483 w499] -> w465
              tunnel: w469 -> [w478 _]
              tunnel: w470 -> [w486 _]
              tunnel: w467 -> [w477 _]
              tunnel: w471 -> [w485 w499]
              tunnel: w464 -> [w482 _]
              frame False {
                n165 = call "ASIA Reserve Pump.vi"("error in (no error)"=w485, "ASIA Pump # In"=w486) -> ("error out"=w481:errorcluster, "ASIA Pump # Out"=w479:i32)  [unwired: 8 in]
                n166 = dll-call lib="C:/Program Files (x86)/Pfizer/FAST/data/AsiaPumpInterface.dll" fn="empty"(error in=w481, "pumpNum"=w479, "channel"=w478, "rate"=w477) -> (error out=w480:errorcluster, "pumpNum"=w476:u32)  [unwired: 5 in, 1 out]
                n167 = call "ASIA Release Pump.vi"("error in (no error)"=w480, "pumpNum"=w476) -> ("error out"=w484:errorcluster)  [unwired: 8 in, 1 out]
                n168 = while {
                  tunnel: w484 -> [w496]
                  tunnel: [w495] -> w483
                  tunnel: w482 -> [w494]
                  i -> [w491]
                  stop <- w488 stop-if-true
                  n169 = call "Pump Status.vi"("ASIA Pump C Settings in"=w494, "error in (no error)"=w496) -> ("PumpStatusCode"=w492:T23, "error out"=w495:errorcluster)  [unwired: 5 in, 7 out]
                  n170 = Wait (ms)(milliseconds to wait=u32 100) -> ()  [unwired: 1 out]
                  n171 = case shown="\"Error\", Default" w492 {
                    tunnel: [FALSE TRUE] -> w489
                    frame "Error", Default {
                    }
                    frame "Empty" {
                    }
                  }
                  n172 = Greater?(x=w491, y=600) -> (0:w487:bool)
                  n173 = Or(x=w489, y=w487) -> (x .or. y?=w488:bool)
                }
              }
              frame True {
              }
            }
          }
          frame Default {
            # "'Default' case only runs if there is a message that isn't defined in any of the other cases.  Output a programming error."
            n174 = Concatenate Strings("The invalid message string " ("string"), w501, " was received in the Pump Module Engine." ("string")) -> (w502:string)
            n175 = Bundle By Name(cluster=errorcluster {"status"=TRUE, "code"=1, "source"=""} ("error constant"), "source"=w502) -> (w500:errorcluster)
          }
        }
        n176 = Unbundle By Name(w17) -> ("State"=w28:T10, "Configuration.Cycle Period"=w26:dbl)
        n177 = call "Error Handler.vi"("error in (no error)"=w34, "Message Queue"=w32) -> ("dup error in"=w33:errorcluster)  [unwired: 8 in, 1 out]
        n178 = case shown="\"Paused\"" w28 {
          tunnel: [w42 1 1] -> w27
          tunnel: w26 -> [w42 _ _]
          frame "Measuring" {
          }
          frame "Idle" {
          }
          frame "Paused" {
          }
        }
        n179 = node-c288(w27) -> ()  [unwired: 1 in, 1 out]
      }
      n180 = node-c288(w12) -> ()  [unwired: 1 out]
    }
    frame Error {
    }
  }
  "error out" <- w3
